vi "Sync SysRef.vi"(0 "fpga reference in":T1[](array[typedef]), 5 "board settings in":T2[](array[typedef]) {"Address Space" items=["VXI/VME A16"=1, "VXI/VME A24"=2, "VXI/VME A32"=3, "VXI/VME A64"=4, "PXI Memory Allocations"=9, "PXI Configuration"=10, "PXI BAR0"=11, "PXI BAR1"=12, "PXI BAR2"=13, "PXI BAR3"=14, "PXI BAR4"=15, "PXI BAR5"=16]}, 11 "error in":errorcluster) -> (4 "fpga reference out":T1[](array[typedef]), 6 "board settings out":T2[](array[typedef]) {"Address Space" items=["VXI/VME A16"=1, "VXI/VME A24"=2, "VXI/VME A32"=3, "VXI/VME A64"=4, "PXI Memory Allocations"=9, "PXI Configuration"=10, "PXI BAR0"=11, "PXI BAR1"=12, "PXI BAR2"=13, "PXI BAR3"=14, "PXI BAR4"=15, "PXI BAR5"=16]}, 15 "error out":errorcluster)   [LabVIEW 2019]
uses:
  <instrlib>/niMmWave/ni3610 and ni3630/controls/public/Main Settings.ctl
  <vilib>/Instr/_visa.llb/VISA Register Access Address Space.ctl
  <instrlib>/niMmWave/ni3610 and ni3630/controls/public/Register Adresses.ctl
  <instrlib>/niMmWave/ni3610 and ni3630/controls/public/Base Card Type.ctl
  <instrlib>/niMmWave/ni3610 and ni3630/controls/private/IQ Card Revision.ctl
  <instrlib>/niMmWave/ni3610 and ni3630/controls/public/Board Capability.ctl
  TypeDefs/Blank FPGA Reference.ctl
  TypeDefs/Shared FPGA Reference.ctl
  <instrlib>/niMmWave/ni3610 and ni3630/controls/public/Trigger Sink.ctl
  <instrlib>/niMmWave/ni3610 and ni3630/controls/public/SPI Cmd.ctl
  <vilib>/Utility/error.llb/Error Cluster From Error Code.vi
  <vilib>/rvi/errors/niLvFpgaAdjustHostInterfaceError.vi
  <vilib>/rvi/interface/nirviReadWriteControl/nirviReadWriteControl.xnode
  <vilib>/rvi/interface/Simulation/niFpgaSimulationCallBeginRW.vi
  <instrlib>/niMmWave/ni3610 and ni3630/ni3610_and_ni3630_Driver_Lib.lvlib
  NiFpgaLv.dll
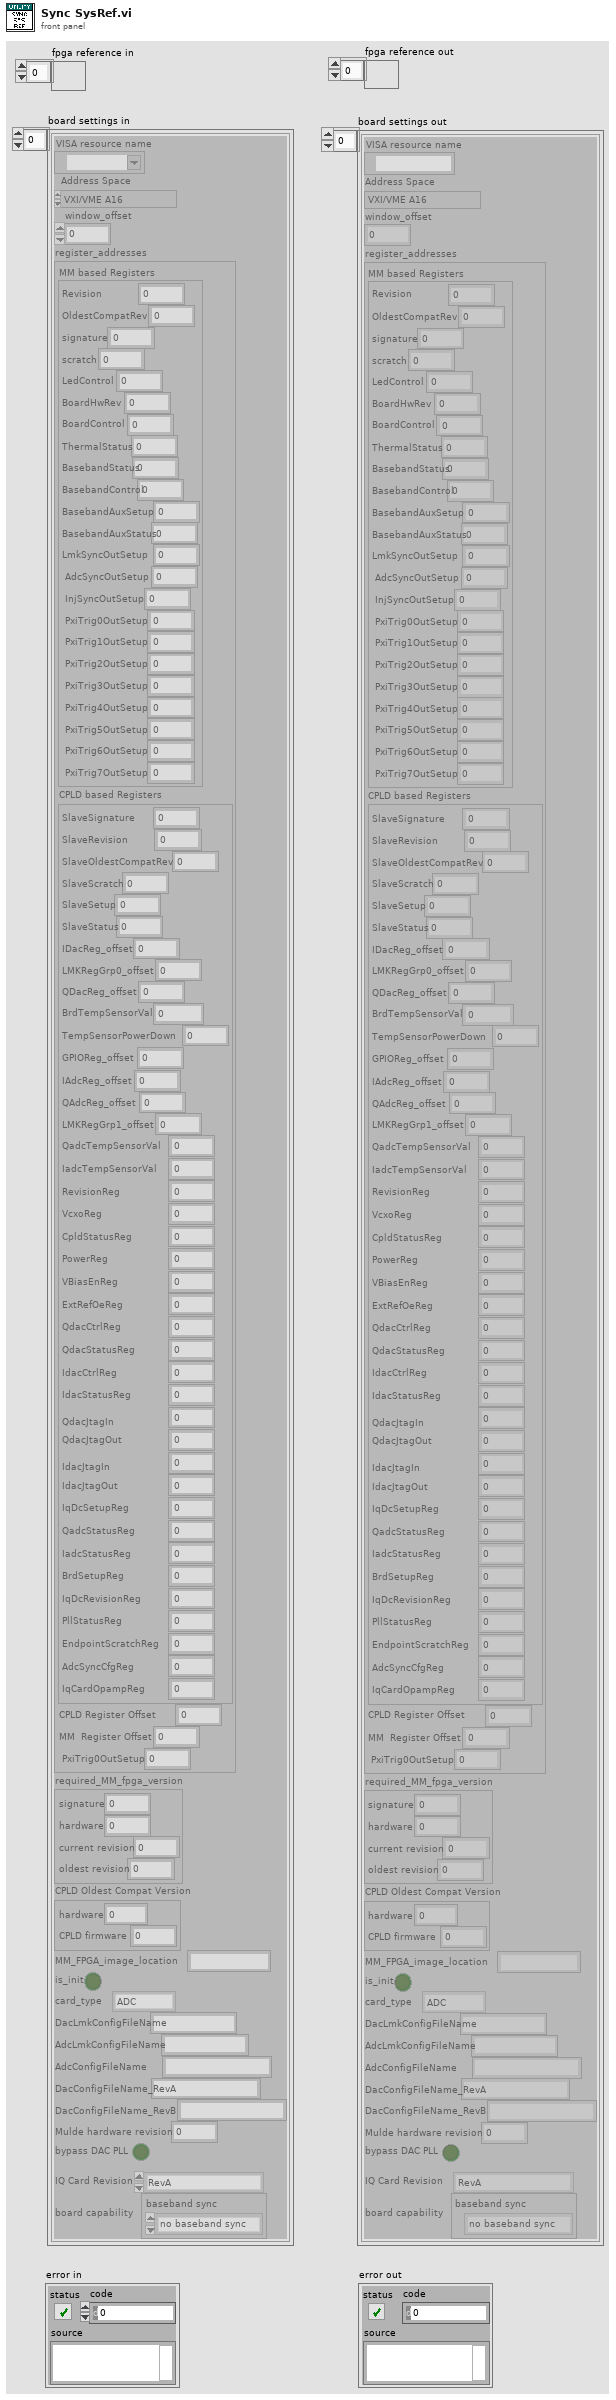
[diagram p1: front panel]
types:
  T1 = typedef "Blank FPGA Reference.ctl" = refnum<k20>
  T2 = typedef "ni3610_and_ni3630_Driver_Lib.lvlib/Main Settings.ctl" = cluster{"VISA resource name":refnum<visa-resource-name>, "Address Space":T3, "window_offset":u32, "register_addresses":T4, "required_MM_fpga_version":cluster{"signature":u32, "hardware":u32, "current revision":u32, "oldest revision":u32}, "CPLD Oldest Compat Version ":cluster{"hardware":u32, "CPLD firmware":u32}, "MM_FPGA_image_location":string, "is_init":bool, "card_type":T5, "DacLmkConfigFileName":string, "AdcLmkConfigFileName":string, "AdcConfigFileName":string, "DacConfigFileName_RevA":string, "DacConfigFileName_RevB":string, "Mulde hardware revision":u8, "bypass DAC PLL\n":bool, "IQ Card Revision":T6, "board capability":T7}
  T3 = typedef "VISA Register Access Address Space.ctl" = u16
  T4 = typedef "ni3610_and_ni3630_Driver_Lib.lvlib/Register Adresses.ctl" = cluster{"MM based Registers":cluster{"Revision":u32, "OldestCompatRev":u32, "signature":u32, "scratch":u32, "LedControl":u32, "BoardHwRev":u32, "BoardControl":u32, "ThermalStatus":u32, "BasebandStatus":u32, "BasebandControl":u32, "BasebandAuxSetup":u32, "BasebandAuxStatus":u32, "LmkSyncOutSetup":u32, " AdcSyncOutSetup":u32, " InjSyncOutSetup":u32, " PxiTrig0OutSetup":u32, " PxiTrig1OutSetup":u32, " PxiTrig2OutSetup":u32, " PxiTrig3OutSetup":u32, " PxiTrig4OutSetup":u32, " PxiTrig5OutSetup":u32, " PxiTrig6OutSetup":u32, " PxiTrig7OutSetup":u32}, "CPLD based Registers":cluster{"SlaveSignature":u32, "SlaveRevision":u32, "SlaveOldestCompatRev":u32, "SlaveScratch":u32, "SlaveSetup":u32, "SlaveStatus":u32, "IDacReg_offset":u32, "LMKRegGrp0_offset":u32, "QDacReg_offset":u32, "BrdTempSensorVal":u32, "TempSensorPowerDown":u32, "GPIOReg_offset":u32, "IAdcReg_offset":u32, "QAdcReg_offset":u32, "LMKRegGrp1_offset":u32, "QadcTempSensorVal":u32, "IadcTempSensorVal":u32, "RevisionReg":u32, "VcxoReg":u32, "CpldStatusReg":u32, "PowerReg":u32, "VBiasEnReg":u32, "ExtRefOeReg":u32, "QdacCtrlReg":u32, "QdacStatusReg":u32, "IdacCtrlReg":u32, "IdacStatusReg":u32, "QdacJtagIn":u32, "QdacJtagOut":u32, "IdacJtagIn":u32, "IdacJtagOut":u32, "IqDcSetupReg":u32, "QadcStatusReg":u32, "IadcStatusReg":u32, "BrdSetupReg":u32, "IqDcRevisionReg":u32, "PllStatusReg":u32, "EndpointScratchReg":u32, "AdcSyncCfgReg":u32, "IqCardOpampReg":u32}, "CPLD Register Offset":u32, "MM  Register Offset":u32, " PxiTrig0OutSetup":u32}
  T5 = typedef "ni3610_and_ni3630_Driver_Lib.lvlib/Base Card Type.ctl" = enum16{"unspecified", "ADC", "DAC"}
  T6 = typedef "ni3610_and_ni3630_Driver_Lib.lvlib/IQ Card Revision.ctl" = enum16{"RevA", "RevB", "RevC", "RevD"}
  T7 = typedef "ni3610_and_ni3630_Driver_Lib.lvlib/Board Capability.ctl" = cluster{"baseband sync":enum16{"no baseband sync", "baseband sync"}}
  T8 = typedef "Shared FPGA Reference.ctl" = refnum<k20>
  T9 = typedef "ni3610_and_ni3630_Driver_Lib.lvlib/Trigger Sink.ctl" = enum16{"LmkSyncOutSetup", "AdcSyncOutSetup", "InjSyncOutSetup"}
  T10 = typedef "ni3610_and_ni3630_Driver_Lib.lvlib/SPI Cmd.ctl" = cluster{"SPI address":u32, "SPI data":u32}
  T11 = cluster{"control":cluster{"measure tdc":bool, "enable measurement":bool, "10 kHz tclk enable":bool, "200 kHz tclk enable":bool, "output enable":bool, "reset":bool, "deassert holdoff":u8, "calibrate":bool, "calibrate width":u8, "tclk trigger enable":bool, "alignment complete":bool}, "tclk parameters":cluster{"rollover count":u16, "rising edge count":u16, "falling edge count":u16}}
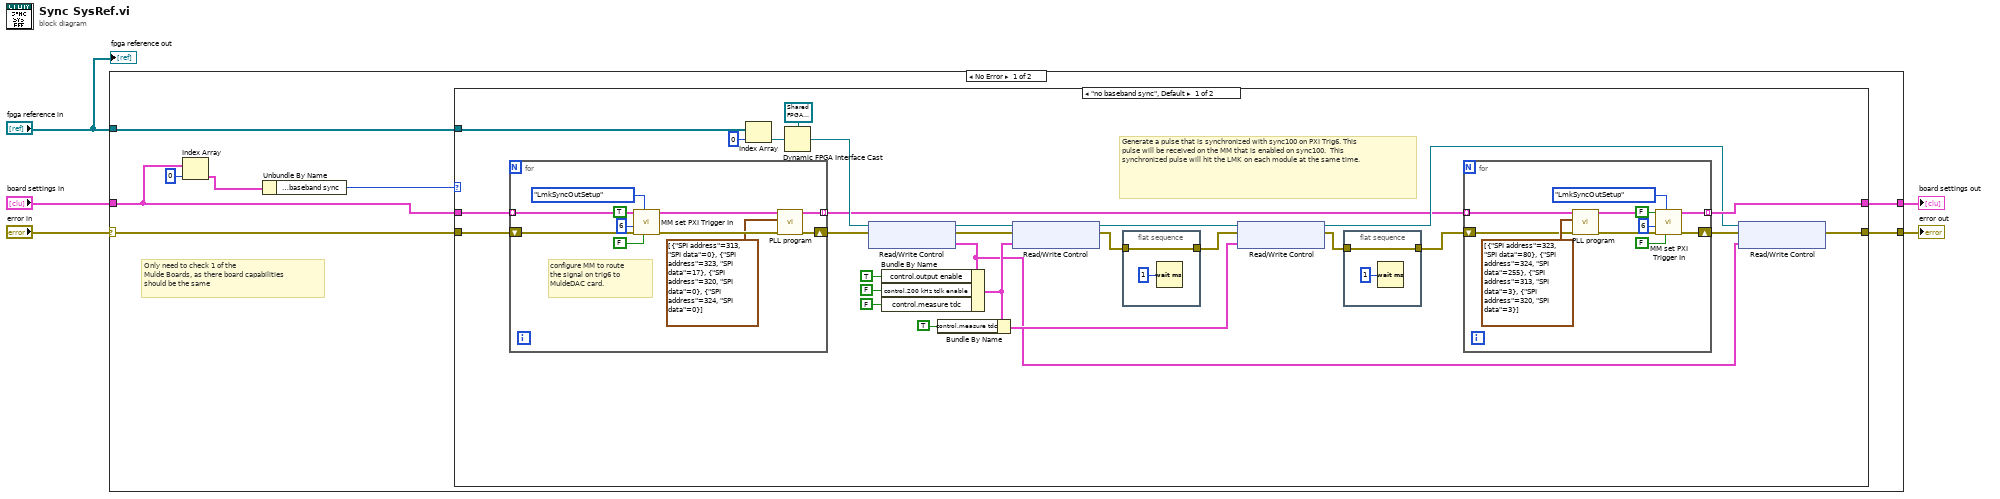
[diagram p0: block diagram]
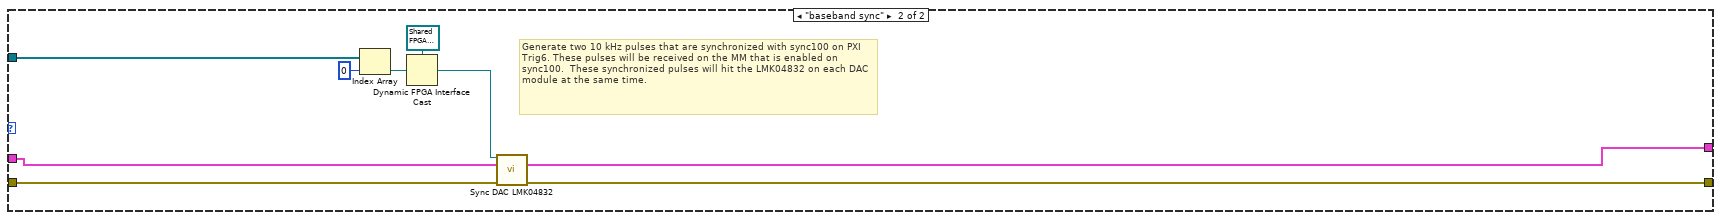
[diagram p2: hidden frame]
diagram:
  n1 = case shown="No Error" "error in" {
    selector: "error in" -> [w7 w77]
    tunnel: "board settings in" -> [w8 w76]
    tunnel: [w13 w77] -> w4
    tunnel: "fpga reference in" -> [w12 _]
    tunnel: [w11 w76] -> w2
    frame No Error {
      # "Only need to check 1 of the \nMulde Boards, as there board capabilities\nshould be the same"
      n2 = Index Array(array=w8, index=0) -> (element=w9:T2)
      n3 = Unbundle By Name(w9) -> ("board capability.baseband sync"=w6:enum16{"no baseband sync", "baseband sync"})
      n4 = case shown="\"no baseband sync\", Default" w6 {
        tunnel: [w40 w75] -> w13
        tunnel: w12 -> [w39 w68]
        tunnel: [w38 w74] -> w11
        tunnel: w7 -> [w15 w72]
        tunnel: w8 -> [w14 w73]
        frame "no baseband sync", Default {
          # "Generate a pulse that is synchronized with sync100 on PXI Trig6. This pulse will be received on the MM that is enabled on sync100.  This synchronized pulse will hit the LMK on each module at the same time."
          n5 = for {
            tunnel: w14 -> [w64] mode=indexing
            shift-right: [w59] -> w33
            shift-left: w15 -> [w63]
            tunnel: [w58] -> w20 mode=indexing
            # "configure MM to route\nthe signal on trig6 to\nMuldeDAC card."
            n6 = call <instrlib>:"MM set PXI Trigger In.vi"("Force Enable"=FALSE, "Trigger Sink"=Trigger_Sink."LmkSyncOutSetup", "error in"=w63, "PXI Trigger Select (0..7)"=u8 6, "Enable Trigger Input"=TRUE, "Board Settings in"=w64) -> ("error out"=w61:errorcluster, "Board Settings out"=w60:T2)  [unwired: 4 in]
            n7 = call <instrlib>:"PLL program.vi"("error in"=w61, "SPI settings array"=T10[] [{"SPI address"=313, "SPI data"=0}, {"SPI address"=323, "SPI data"=17}, {"SPI address"=320, "SPI data"=0}, {"SPI address"=324, "SPI data"=0}], "Board Settings in"=w60) -> ("error out"=w59:errorcluster, "Board Settings out"=w58:T2)  [unwired: 7 in]
          }
          n8 = Index Array(array=w39, index=0) -> (element=w29:T1)
          n9 = Dynamic FPGA Interface Cast(Session In=T8 refnum ("fpga reference"), Type=w29) -> (Session Out=w31:T8)
          n10 = xnode "Read/Write Control"("FPGA VI Reference In"=w31, "error in"=w33) -> ("FPGA VI Reference Out"=w36:T8, "error out"=w37:errorcluster, "sync.parameters"=w24:T11)
          n11 = Bundle By Name(cluster=w24, "control.output enable"=TRUE, "control.200 kHz tclk enable"=FALSE ("control.pulse injection"), "control.measure tdc"=FALSE ("control.measure")) -> (w25:T11)
          n12 = Bundle By Name(cluster=w25, "control.measure tdc"=TRUE ("control.measure")) -> (w27:T11)
          n13 = xnode "Read/Write Control"("FPGA VI Reference In"=w36, "error in"=w37, "sync.parameters"=w25) -> ("FPGA VI Reference Out"=w19:T8, "error out"=w18:errorcluster)
          n14 = flat-sequence {
            tunnel: [w43] -> w17
            tunnel: w18 -> [w43]
            frame #0 {
              n15 = Wait (ms)(milliseconds to wait=u32 1) -> ()  [unwired: 1 out]
            }
          }
          n16 = xnode "Read/Write Control"("FPGA VI Reference In"=w19, "error in"=w17, "sync.parameters"=w27) -> ("FPGA VI Reference Out"=w21:T8, "error out"=w16:errorcluster)
          n17 = flat-sequence {
            tunnel: [w41] -> w22
            tunnel: w16 -> [w41]
            frame #0 {
              n18 = Wait (ms)(milliseconds to wait=u32 1) -> ()  [unwired: 1 out]
            }
          }
          n19 = for {
            tunnel: w20 -> [w51] mode=indexing
            shift-right: [w46] -> w26
            shift-left: w22 -> [w50]
            tunnel: [w47] -> w38 mode=indexing
            n20 = call <instrlib>:"PLL program.vi"("error in"=w50, "SPI settings array"=T10[] [{"SPI address"=323, "SPI data"=80}, {"SPI address"=324, "SPI data"=255}, {"SPI address"=313, "SPI data"=3}, {"SPI address"=320, "SPI data"=3}], "Board Settings in"=w51) -> ("error out"=w49:errorcluster, "Board Settings out"=w48:T2)  [unwired: 7 in]
            n21 = call <instrlib>:"MM set PXI Trigger In.vi"("Force Enable"=FALSE, "Trigger Sink"=Trigger_Sink."LmkSyncOutSetup", "error in"=w49, "PXI Trigger Select (0..7)"=u8 6, "Enable Trigger Input"=FALSE, "Board Settings in"=w48) -> ("error out"=w46:errorcluster, "Board Settings out"=w47:T2)  [unwired: 4 in]
          }
          n22 = xnode "Read/Write Control"("FPGA VI Reference In"=w21, "error in"=w26, "sync.parameters"=w24) -> ("error out"=w40:errorcluster)  [unwired: 1 out]
        }
        frame "baseband sync" {
          # "Generate two 10 kHz pulses that are synchronized with sync100 on PXI Trig6. These pulses will be received on the MM that is enabled on sync100.  These synchronized pulses will hit the LMK04832 on each DAC module at the same time."
          n23 = Index Array(array=w68, index=0) -> (element=w69:T1)
          n24 = Dynamic FPGA Interface Cast(Session In=T8 refnum ("fpga reference"), Type=w69) -> (Session Out=w67:T8)
          n25 = call "Sync DAC LMK04832.vi"("fpga reference in"=w67, "board settings in"=w73, "error in"=w72) -> ("board settings out"=w74:T2[], "error out"=w75:errorcluster)  [unwired: 11 in]
        }
      }
    }
    frame Error {
    }
  }
  "error out" <- w4
  "board settings out" <- w2
  "fpga reference out" <- "fpga reference in"
